vi "_Delete Text from HTML.vi"(0 "HTML File Path":path, 5 "Text Before Delete":string, 9 "Text After Delete":string, 11 "error in":errorcluster) -> (4 "HTML File Path out":path, 15 "error out":errorcluster)   [LabVIEW 2012]
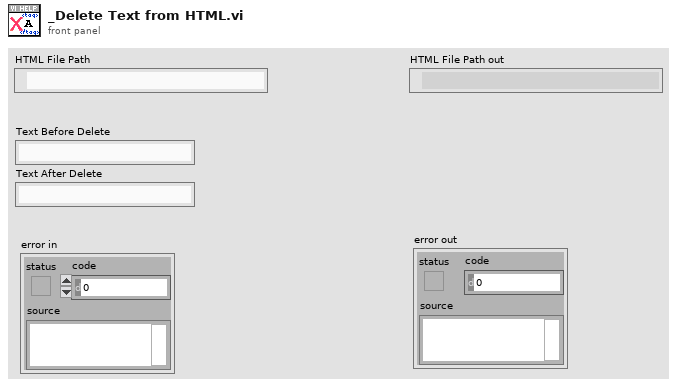
[diagram p1: front panel]
types:
  T1 = enum16{"open", "replace", "create", "open or create", "replace or create", "replace or create with confirmation"}
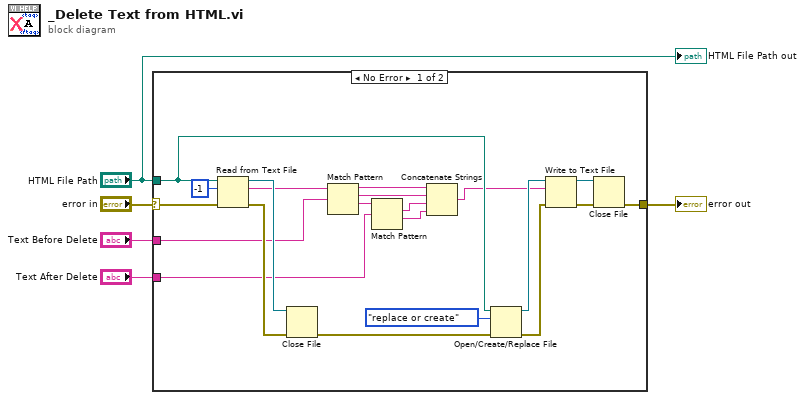
[diagram p0: block diagram]
diagram:
  n1 = case shown="No Error" "error in" {
    selector: "error in" -> [w6 w27]
    tunnel: "HTML File Path" -> [w19 _]
    tunnel: [w18 w27] -> w4
    tunnel: "Text After Delete" -> [w15 _]
    tunnel: "Text Before Delete" -> [w7 _]
    frame No Error {
      n2 = Read from Text File(file (use dialog)=w19, count=-1, error in=w6) -> (refnum out=w22:refnum<file>, text=w10:string, error out=w23:errorcluster)  [unwired: 1 in, 1 out]
      n3 = Close File(refnum=w22, error in=w23) -> (error out=w8:errorcluster)  [unwired: 1 out]
      n4 = Match Pattern(string=w10, regular expression=w7) -> (before substring=w14:string, match substring=w13:string, after substring=w16:string)  [unwired: 1 in, 1 out]
      n5 = Match Pattern(string=w16, regular expression=w15) -> (match substring=w12:string, after substring=w11:string)  [unwired: 1 in, 2 out]
      n6 = Concatenate Strings(w14, w13, w12, w11) -> (w9:string)
      n7 = Open/Create/Replace File(file path (use dialog)=w19, error in=w8, operation (0:open)=T1."replace or create") -> (refnum out=w21:refnum<file>, error out=w20:errorcluster)  [unwired: 3 in, 1 out]
      n8 = Write to Text File(file (use dialog)=w21, text=w9, error in=w20) -> (refnum out=w26:refnum<file>, error out=w25:errorcluster)  [unwired: 1 in, 1 out]
      n9 = Close File(refnum=w26, error in=w25) -> (error out=w18:errorcluster)  [unwired: 1 out]
    }
    frame Error {
    }
  }
  "error out" <- w4
  "HTML File Path out" <- "HTML File Path"
